vi "UdpServer.vi"() -> ()   [LabVIEW 2012]
panel:
  out "error out":errorcluster
  out "String":string
  out "Waveform Chart":dbl(graph)
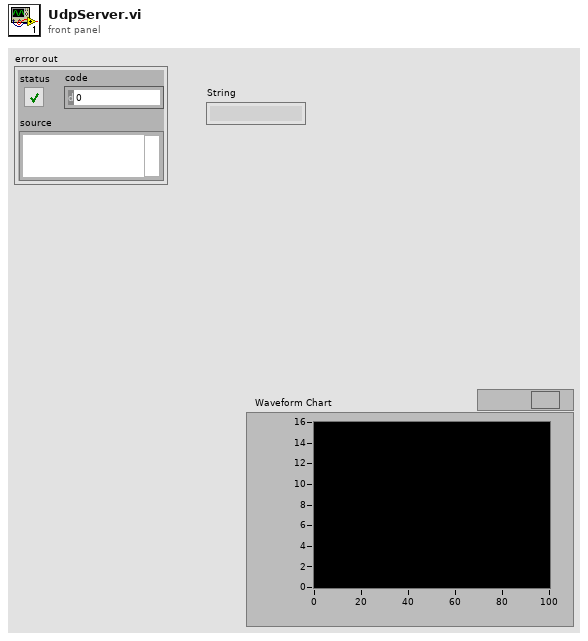
[diagram p1: front panel]
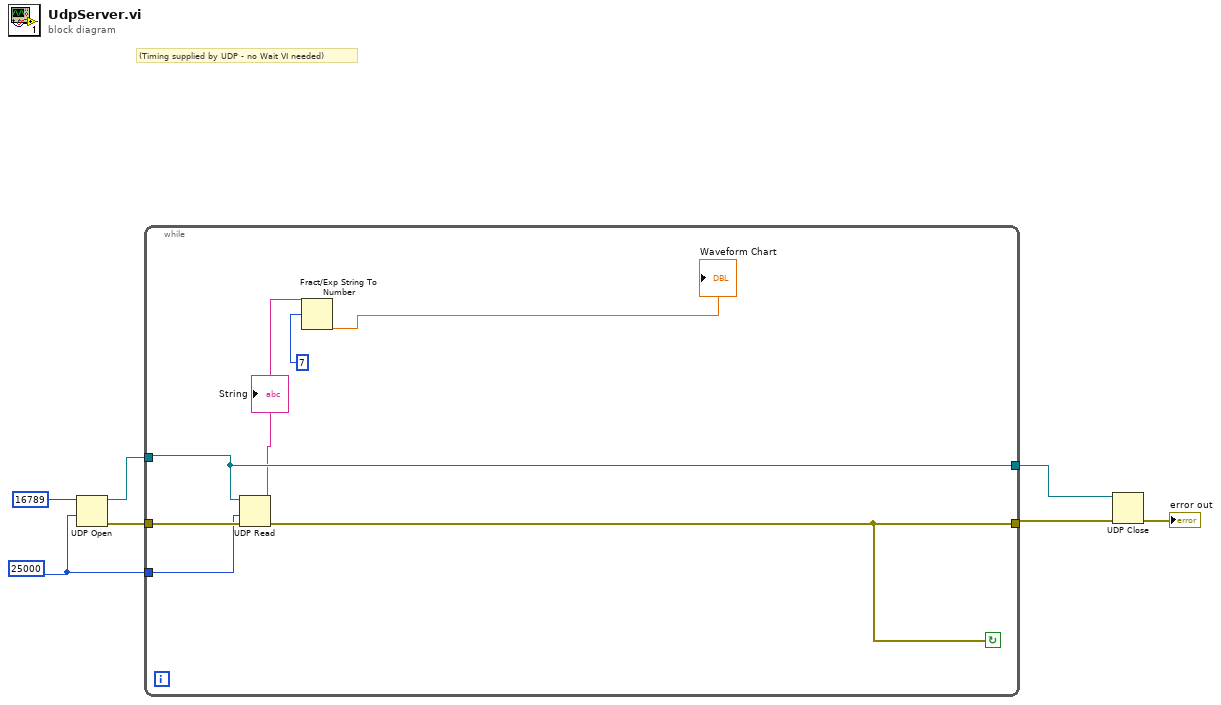
[diagram p0: block diagram]
diagram:
  w4 = 25000 ("timeout ms (25000)")
  # "(Timing supplied by UDP - no Wait VI needed)"
  n1 = UDP Open(9:w4, 11:u16 16789 ("port")) -> (port=w7:refnum<k16>, 0:w6:errorcluster)  [unwired: 3 in, 1 out]
  n2 = while {
    tunnel: w7 -> [w12]
    tunnel: w6 -> [w14]
    tunnel: w4 -> [w13]
    tunnel: [w8] -> w2
    tunnel: [w12] -> w1
    stop <- w8 continue-if-true
    n3 = UDP Read(connection ID=w12, timeout ms (25000)=w13, 8:w14) -> (data out=w10:string, error out=w8:errorcluster)  [unwired: 1 in, 3 out]
    "String" <- w10
    n4 = Fract/Exp String To Number(string=w10, offset=7 ("timeout ms (25000)")) -> (number=→"Waveform Chart":dbl)  [unwired: 2 in, 1 out]
  }
  n5 = UDP Close(connection ID=w1, 8:w2) -> (error out=→"error out":errorcluster)  [unwired: 1 out]
